vi "Switch Solenoid Feedthrough.vi"(8 "error in (no error)":errorcluster, 10 "Only Turn On (F)":bool, 11 "Feeder Actor.lvlib:Feeder.lvclass":refnum<class "Feeder.lvclass">) -> (0 "error out":errorcluster, 3 "Actor out":refnum<class "Actor.lvclass">)   [LabVIEW 2018, in "Feeder Actor.lvlib" / "Feeder.lvclass"]
uses:
  Feeder.lvclass
  <vilib>/ActorFramework/Actor/Actor.lvclass
  C:/Program Files/National Instruments/LabVIEW 2018/vi.lib/ActorFramework/Actor/Actor.lvclass
  Feeder.lvclass/Feeder.ctl
  Solenoid Messages/Switch Solenoid Msg/Switch Solenoid Msg.lvclass/Switch Solenoid Msg.ctl
  <vilib>/ActorFramework/Message Enqueuer/Message Enqueuer.lvclass/Message Enqueuer.ctl
  Solenoid Messages/Set Solonoid Msg/Set Solonoid Msg.lvclass/Set Solonoid Msg.ctl
  <vilib>/ActorFramework/Message Enqueuer/Enqueue.vi
  Solenoid Messages/Switch Solenoid Msg/Switch Solenoid Msg.lvclass
  C:/Program Files/National Instruments/LabVIEW 2018/vi.lib/ActorFramework/Message/Message.lvclass
  Solenoid Messages/Set Solonoid Msg/Set Solonoid Msg.lvclass
  <vilib>/ActorFramework/Message Priority Queue/Priority Enqueue.vi
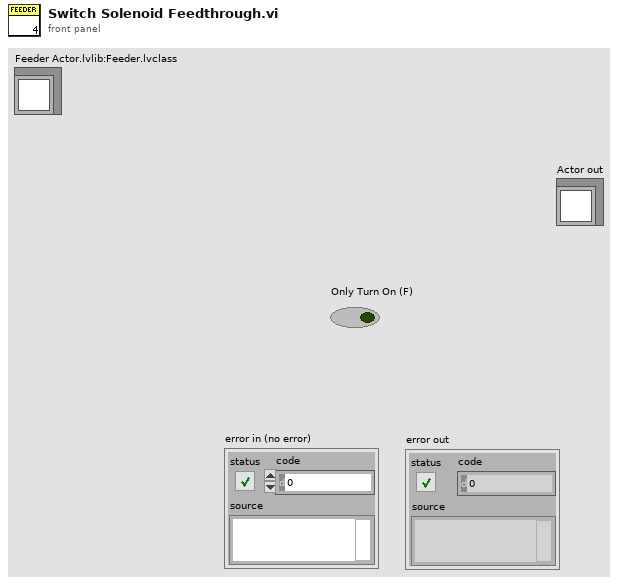
[diagram p1: front panel]
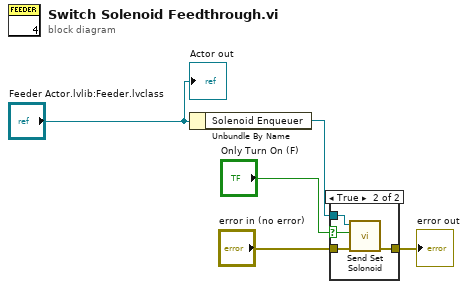
[diagram p0: block diagram]
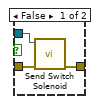
[diagram p2: hidden frame]
diagram:
  n1 = Unbundle By Name("Feeder Actor.lvlib:Feeder.lvclass") -> ("Solenoid Enqueuer"=w5:refnum<class "Message Enqueuer.lvclass">)
  n2 = case shown="True" "Only Turn On (F)" {
    selector: "Only Turn On (F)" -> [_ w11]
    tunnel: w5 -> [w6 w12]
    tunnel: "error in (no error)" -> [w8 w10]
    tunnel: [w7 w9] -> w3
    frame False {
      n3 = call "Send Switch Solenoid.vi"("error in (no error)"=w8, "Message Enqueuer in"=w6) -> ("error out"=w7:errorcluster)  [unwired: 8 in, 1 out]
    }
    frame True {
      n4 = call "Send Set Solonoid.vi"("error in (no error)"=w10, "State"=w11, "Message Enqueuer"=w12) -> ("error out"=w9:errorcluster)  [unwired: 7 in, 1 out]
    }
  }
  "error out" <- w3
  "Actor out" <- "Feeder Actor.lvlib:Feeder.lvclass"
